vi "Parse Query.vi"(8 "error in (no error)":errorcluster, 9 "Query":string, 10 "Database In":refnum<class "Database Platform.lvclass">) -> (0 "error out":errorcluster, 2 "Database":refnum<class "Database Platform.lvclass">, 3 "Query Builder out":refnum<class "Query Builder.lvclass">)   [LabVIEW 2020, in "Conditu2.lvlib" / "Query Builder.lvclass"]
uses:
  Query Builder.lvclass
  Database Platform/Database Platform.lvclass
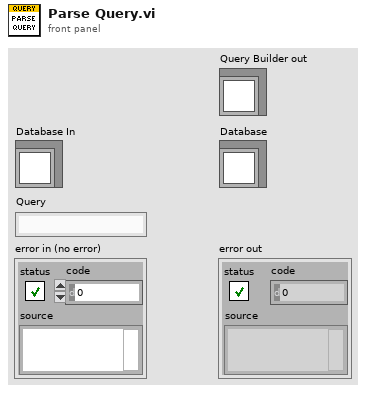
[diagram p1: front panel]
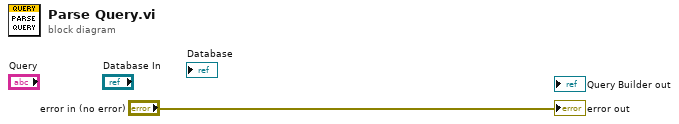
[diagram p0: block diagram]
diagram:
  "error out" <- "error in (no error)"
